vi "Lorentzian model function.vi"(3 "output control":T1, 4 "data":variant, 5 "X":dbl[](array[numeric]), 6 "a":dbl[](array[numeric])) -> (0 "error out":errorcluster, 1 "f'(X,a)":dbl[][](array[numeric]), 2 "f(X,a)":dbl[](array[numeric]))   [LabVIEW 2016]
doc: "This template is the starting point for creating a model function to be passed to the Nonlinear Curve Fit.vi."
uses:
  <vilib>/gmath/NumericalOptimization/LM_output select.ctl
  <vilib>/gmath/NI_Gmath.lvlib
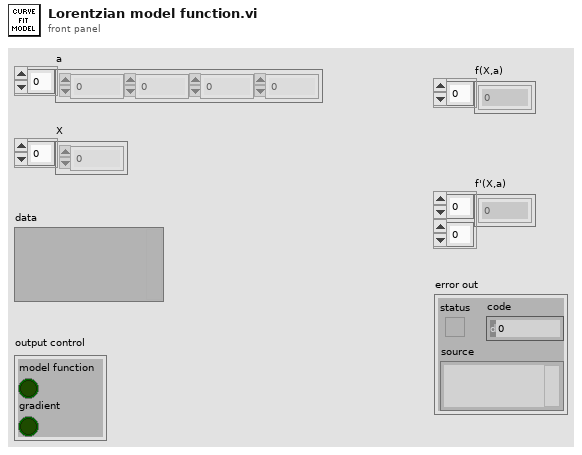
[diagram p1: front panel]
types:
  T1 = typedef "NI_Gmath.lvlib/LM_output select.ctl" = cluster{"model function":bool, "gradient":bool}
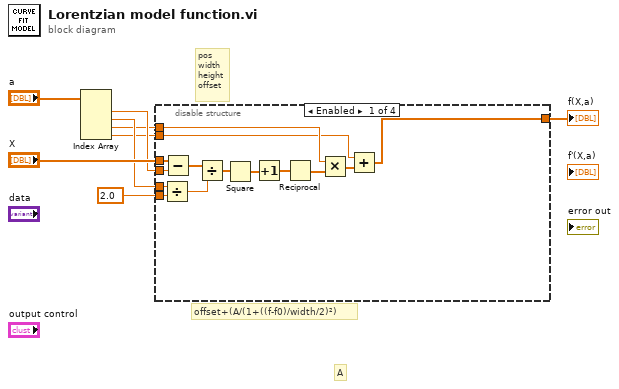
[diagram p0: block diagram]
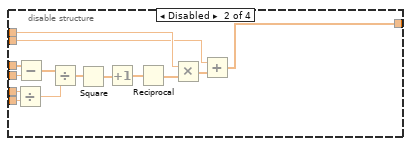
[diagram p2: hidden frame]
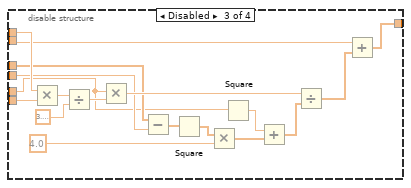
[diagram p3: hidden frame]
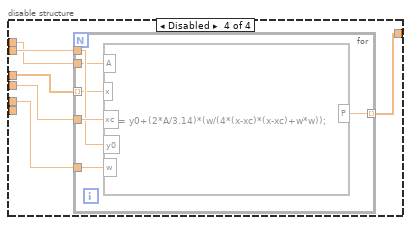
[diagram p4: hidden frame]
diagram:
  # "A"
  # "offset+(A/(1+((f-f0)/width/2)²)"
  # "pos\nwidth\nheight\noffset"
  n1 = Index Array(array="a") -> (element #1=w5:dbl, element #2=w4:dbl, element #3=w3:dbl, element #4=w2:dbl)  [unwired: 4 in]
  n2 = disable-structure shown="Enabled" {
    disable-tunnel: 2.0 ("y") -> [w22 w36 w54 _]
    disable-tunnel: "X" -> [w17 w31 w47 w55]
    disable-tunnel: w5 -> [w16 w30 w46 w60]
    disable-tunnel: w4 -> [w15 w29 w40 w59]
    disable-tunnel: w3 -> [w12 w26 w53 w57]
    disable-tunnel: w2 -> [w10 w24 w39 w58]
    disable-tunnel: [w9 w23 w37 w56] -> w1
    frame Enabled {
      n3 = Divide(x=w15, y=w22) -> (x/y=w14:dbl)
      n4 = Subtract(x=w17, y=w16) -> (x-y=w18:dbl[])
      n5 = Divide(x=w18, y=w14) -> (x/y=w21:dbl[])
      n6 = Square(x=w21) -> (x^2=w20:dbl[])
      n7 = Increment(x=w20) -> (x+1=w19:dbl[])
      n8 = Reciprocal(x=w19) -> (1/x=w13:dbl[])
      n9 = Multiply(x=w12, y=w13) -> (x*y=w11:dbl[])
      n10 = Add(x=w10, y=w11) -> (x+y=w9:dbl[])
    }
    frame Disabled {
      n11 = Divide(x=w29, y=w36) -> (x/y=w28:dbl)
      n12 = Subtract(x=w31, y=w30) -> (x-y=w32:dbl[])
      n13 = Divide(x=w32, y=w28) -> (x/y=w35:dbl[])
      n14 = Square(x=w35) -> (x^2=w34:dbl[])
      n15 = Increment(x=w34) -> (x+1=w33:dbl[])
      n16 = Reciprocal(x=w33) -> (1/x=w27:dbl[])
      n17 = Multiply(x=w26, y=w27) -> (x*y=w25:dbl[])
      n18 = Add(x=w24, y=w25) -> (x+y=w23:dbl[])
    }
    frame Disabled {
      n19 = Multiply(x=w53, y=w54) -> (x*y=w52:dbl)
      n20 = Divide(x=w52, y=3.141592653589793) -> (x/y=w50:dbl)
      n21 = Multiply(x=w40, y=w50) -> (x*y=w49:dbl)
      n22 = Subtract(x=w47, y=w46) -> (x-y=w45:dbl[])
      n23 = Square(x=w45) -> (x^2=w44:dbl[])
      n24 = Multiply(x=w44, y=4.0) -> (x*y=w43:dbl[])
      n25 = Square(x=w40) -> (x^2=w42:dbl)
      n26 = Add(x=w42, y=w43) -> (x+y=w41:dbl[])
      n27 = Divide(x=w49, y=w41) -> (x/y=w38:dbl[])
      n28 = Add(x=w39, y=w38) -> (x+y=w37:dbl[])
    }
    frame Disabled {
      n29 = for {
        tunnel: w60 -> [w66]
        tunnel: w59 -> [w65]
        tunnel: w58 -> [w64]
        tunnel: w57 -> [w63]
        tunnel: [w62] -> w56 mode=indexing
        tunnel: w55 -> [w61] mode=indexing
        n30 = formula code="P= y0+(2*A/3.14)*(w/(4*(x-xc)*(x-xc)+w*w));"("A"=w63, "w"=w65, "xc"=w66, "y0"=w64, "x"=w61) -> ("P"=w62:dbl)
      }
    }
  }
  "f(X,a)" <- w1
